vi "Turn Smother.vi"(2 "Ignore Deceleration":bool, 3 "Ignore Acceleration":bool, 4 "input cluster":T5={"Trajectory Data"=[], "Updated Waypoints"=[], {"Sample Period (s)"=0.0, "Limits"={"Velocity (fps)"=6.0, "Accel (fps^2)"=15.0, "Jerk (fps^3)"=150.0, "StoopidFast (fps)"=6.0}, "Conditions"={"vInitial (fps)"=0.0, "vFinal (fps)"=0.0}, "Angular Accelerations"={"Angular \nAccelerations"=[], "Override Limits?"=[]}}, "Array"=[]} {"?"."Limits"."StoopidFast (fps)" min=0.0; "?"."Limits"."Jerk (fps^3)" min=0.0 step=1.0; "?"."Limits"."Accel (fps^2)" min=0.0; "?"."Limits"."Velocity (fps)" min=0.0}) -> (0 "Velocities":dbl[](array[numeric]), 1 "Angular Accelerations":T1)   [LabVIEW 2019]
uses:
  Limits.ctl
  Command Stuff/Single Cmd Info.ctl
  <vilib>/picture/picture.llb/imagedata.ctl
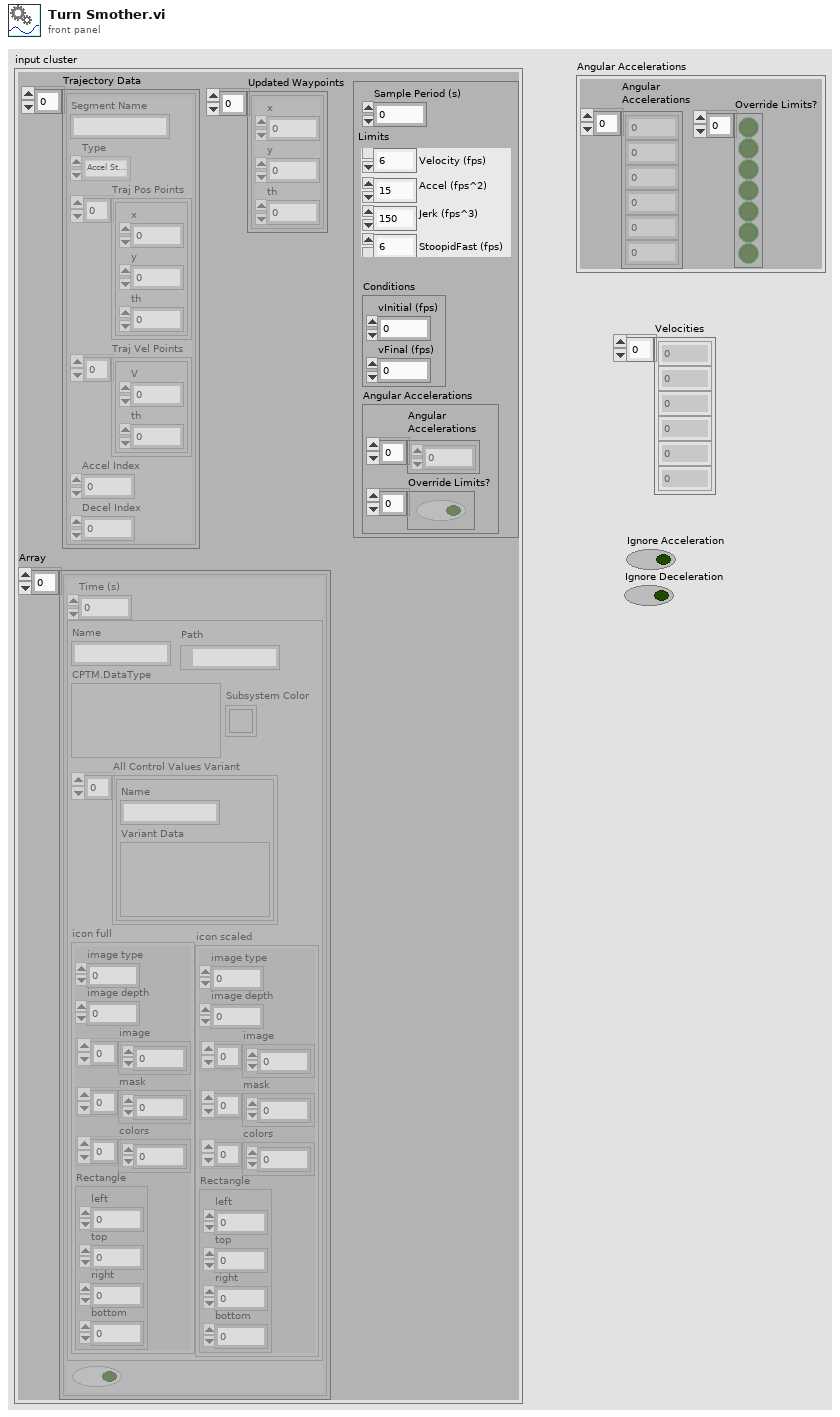
[diagram p1: front panel]
types:
  T1 = cluster{"Angular \nAccelerations":dbl[], "Override Limits?":bool[]}
  T2 = typedef "Limits.ctl" = cluster{"Velocity (fps)":dbl, "Accel (fps^2)":dbl, "Jerk (fps^3)":dbl, "StoopidFast (fps)":dbl}
  T3 = typedef "Single Cmd Info.ctl" = cluster{"Name":string, "CPTM.DataType":variant, "All Control Values Variant":cluster{"Name":string, "Variant Data":variant}[], "icon full":T4, "icon scaled":T4, "Path":path, "Subsystem Color":u32}
  T4 = typedef "imagedata.ctl" = cluster{"image type":i32, "image depth":i32, "image":u8[], "mask":u8[], "colors":u32[], "Rectangle":cluster{"left":i16, "top":i16, "right":i16, "bottom":i16}}
  T5 = cluster{"Trajectory Data":cluster{"Segment Name":string, "Type":enum16{"Accel Straight", "Const Straight", "Blend", "Circle"}, "Traj Pos Points":cluster{"x":dbl, "y":dbl, "th":dbl}[], "Traj Vel Points":cluster{"V":dbl, "th":dbl}[], "Accel Index":i32, "Decel Index":i32}[], "Updated Waypoints":cluster{"x":dbl, "y":dbl, "th":dbl}[], cluster{"Sample Period (s)":dbl, "Limits":T2, "Conditions":cluster{"vInitial (fps)":dbl, "vFinal (fps)":dbl}, "Angular Accelerations":cluster{"Angular \nAccelerations":dbl[], "Override Limits?":bool[]}}, "Array":cluster{"Time (s)":dbl, T3, bool}[]}
  T6 = cluster{"Segment Name":string, "Type":enum16{"Accel Straight", "Const Straight", "Blend", "Circle"}, "Traj Pos Points":cluster{"x":dbl, "y":dbl, "th":dbl}[], "Traj Vel Points":cluster{"V":dbl, "th":dbl}[], "Accel Index":i32, "Decel Index":i32}[]
  T7 = cluster{"Sample Period (s)":dbl, "Limits":T2, "Conditions":cluster{"vInitial (fps)":dbl, "vFinal (fps)":dbl}, "Angular Accelerations":cluster{"Angular \nAccelerations":dbl[], "Override Limits?":bool[]}}
  T8 = cluster{"vInitial (fps)":dbl, "vFinal (fps)":dbl}
  T9 = cluster{"Segment Name":string, "Type":enum16{"Accel Straight", "Const Straight", "Blend", "Circle"}, "Traj Pos Points":cluster{"x":dbl, "y":dbl, "th":dbl}[], "Traj Vel Points":cluster{"V":dbl, "th":dbl}[], "Accel Index":i32, "Decel Index":i32}
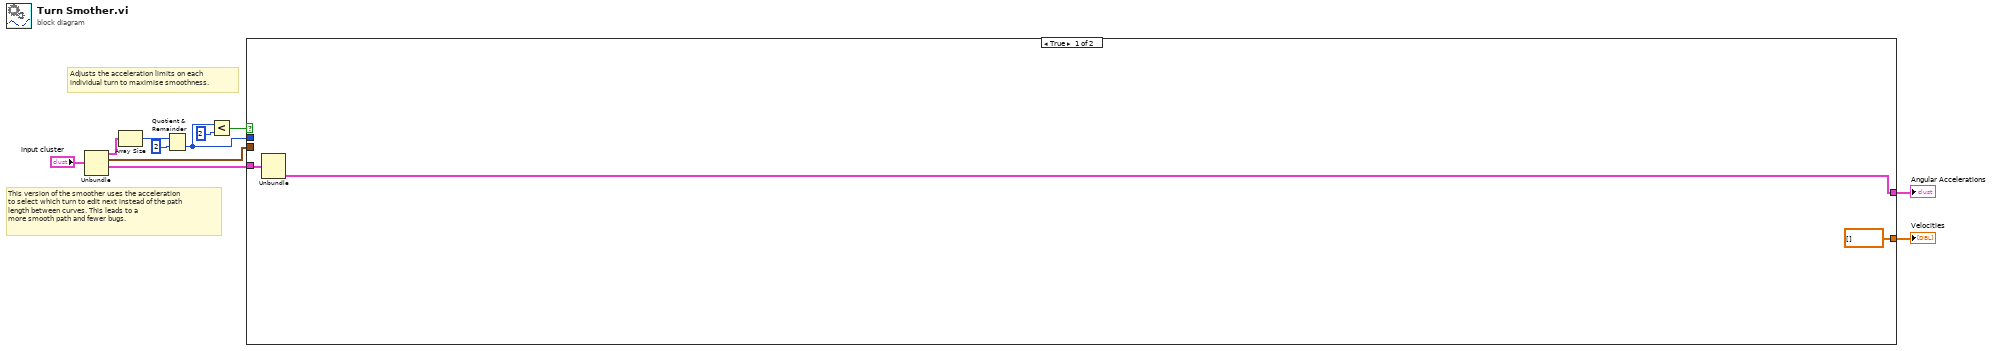
[diagram p0: block diagram]
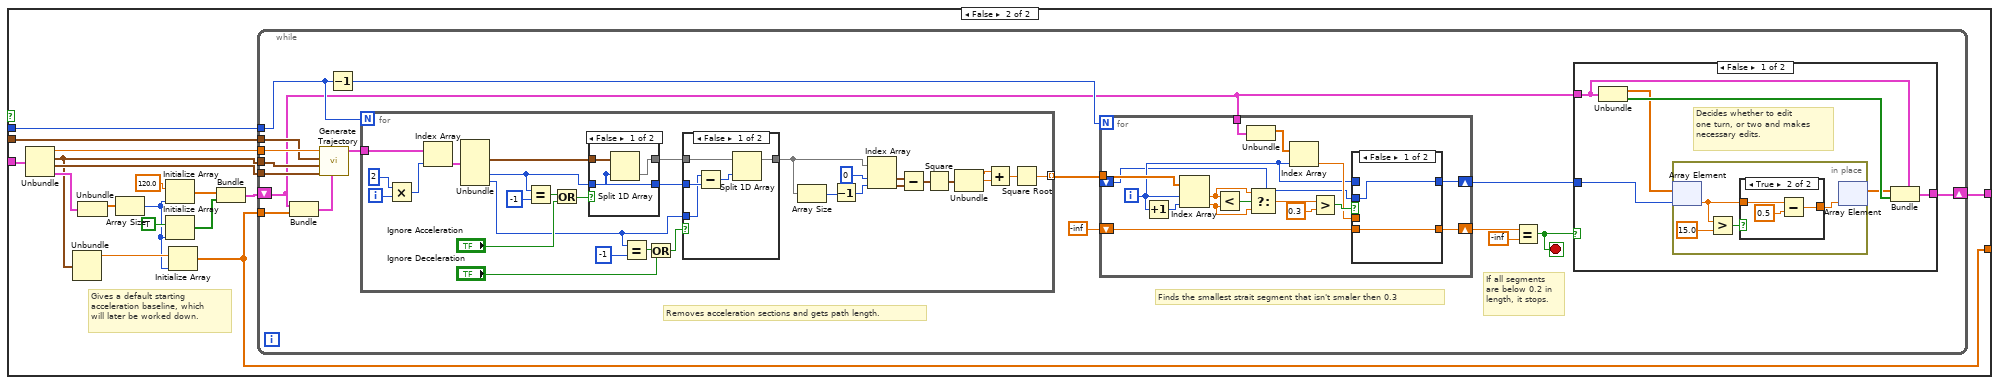
[diagram p2: hidden frame]
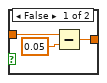
[diagram p3: hidden frame]
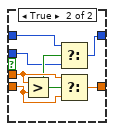
[diagram p7: hidden frame]
diagram:
  # "This version of the smoother uses the acceleration\nto select which turn to edit next instead of the path \nlength between curves. This leads to a \nmore smooth path and fewer bugs."
  # "Adjusts the acceleration limits on each \nindividual turn to maximise smoothness."
  n1 = Unbundle("input cluster") -> ("Trajectory Data"=w4:T6, "Updated Waypoints"=w3:cluster{"x":dbl, "y":dbl, "th":dbl}[], w5:T7)  [unwired: 1 out]
  n2 = Array Size(array=w4) -> (size(s)=w11:i32)
  n3 = Quotient & Remainder(x=w11, y=2) -> (floor(x/y)=w7:i32)  [unwired: 1 out]
  n4 = Less?(x=w7, y=2) -> (x < y?=w6:bool)
  n5 = case shown="True" w6 {
    tunnel: w7 -> [_ w29]
    tunnel: [w14 w28] -> w2
    tunnel: w5 -> [w13 w27]
    tunnel: w3 -> [_ w25]
    tunnel: [dbl[] [] w15] -> w1
    frame True {
      n6 = Unbundle(w13) -> ("Angular Accelerations"=w14:T1)  [unwired: 3 out]
    }
    frame False {
      # "Gives a default starting \nacceleration baseline, which\nwill later be worked down."
      n7 = Unbundle(w27) -> ("Sample Period (s)"=w26:dbl, "Limits"=w22:T2, "Conditions"=w24:T8, "Angular Accelerations"=w31:T1)
      n8 = Unbundle(w22) -> ("Velocity (fps)"=w23:dbl)  [unwired: 3 out]
      n9 = Unbundle(w31) -> ("Angular \nAccelerations"=w16:dbl[])  [unwired: 1 out]
      n10 = Array Size(array=w16) -> (size(s)=w18:i32)
      n11 = Initialize Array(120.0, w18) -> (w17:dbl[])
      n12 = Initialize Array(TRUE, w18) -> (w20:bool[])
      n13 = Initialize Array(w23, w18) -> (w15:dbl[])
      n14 = Bundle(w17, w20) -> (w30:cluster{dbl[], bool[]})  [unwired: 1 in]
      n15 = while {
        shift-right: [w46] -> w28
        shift-left: w30 -> [w34]
        tunnel: w29 -> [w43]
        tunnel: w26 -> [w41]
        tunnel: w25 -> [w40]
        tunnel: w22 -> [w39]
        tunnel: w24 -> [w38]
        tunnel: w15 -> [w33]
        stop <- w48 stop-if-true
        # "If all segments\nare below 0.2 in\nlength, it stops."
        # "Removes acceleration sections and gets path length."
        # "Finds the smallest strait segment that isn't smaler then 0.3"
        n16 = Bundle(w34, w33) -> (w32:cluster{cluster{dbl[], bool[]}, dbl[]})  [unwired: 1 in]
        n17 = call "Generate Trajectory.vi"("Overrides"=w32, "Conditions"=w38, "Limits"=w39, "WayPoints"=w40, "Sample Period (s)"=w41) -> ("Trajectory Data"=w42:T6)  [unwired: 2 in, 4 out]
        n18 = Decrement(x=w43) -> (x-1=w44:i32)
        n19 = for {
          N: w43 -> [_]
          tunnel: w42 -> [w93]
          tunnel: [w83] -> w45 mode=indexing
          i -> [w95]
          n20 = Multiply(x=2, y=w95) -> (x*y=w92:i32)
          n21 = Index Array(array=w93, index=w92) -> (element=w91:T9)
          n22 = Unbundle(w91) -> ("Traj Pos Points"=w84:cluster{"x":dbl, "y":dbl, "th":dbl}[], "Accel Index"=w80:i32, "Decel Index"=w73:i32)  [unwired: 3 out]
          n23 = Equal?(x=w80, y=-1) -> (x = y?=w81:bool)
          n24 = Or(x=w81, y="Ignore Acceleration") -> (x .or. y?=w79:bool)
          n25 = case shown="False" w79 {
            tunnel: w84 -> [w104 w105]
            tunnel: [w103 w105] -> w90
            tunnel: [w102 _] -> w89
            tunnel: w80 -> [w102 _]
            frame False {
              n26 = Split 1D Array(array=w104, index=w102) -> (second subarray=w103:cluster{"x":dbl, "y":dbl, "th":dbl}[])  [unwired: 1 out]
            }
            frame True {
            }
          }
          n27 = Equal?(x=w73, y=-1) -> (x = y?=w76:bool)
          n28 = Or(x=w76, y="Ignore Deceleration") -> (x .or. y?=w74:bool)
          n29 = case shown="False" w74 {
            tunnel: w90 -> [w100 w101]
            tunnel: [w99 w101] -> w87
            tunnel: w89 -> [w98 _]
            tunnel: w73 -> [w96 _]
            frame False {
              n30 = Subtract(x=w96, y=w98) -> (x-y=w97:i32)
              n31 = Split 1D Array(array=w100, index=w97) -> (first subarray=w99:cluster{"x":dbl, "y":dbl, "th":dbl}[])  [unwired: 1 out]
            }
            frame True {
            }
          }
          n32 = Array Size(array=w87) -> (size(s)=w86:i32)
          n33 = Decrement(x=w86) -> (x-1=w85:i32)
          n34 = Index Array(array=w87, index #1=0 ("index"), index #2=w85) -> (element #1=w72:cluster{"x":dbl, "y":dbl, "th":dbl}, element #2=w71:cluster{"x":dbl, "y":dbl, "th":dbl})
          n35 = Subtract(x=w72, y=w71) -> (x-y=w70:cluster{"x":dbl, "y":dbl, "th":dbl})
          n36 = Square(x=w70) -> (x^2=w69:cluster{"x":dbl, "y":dbl, "th":dbl})
          n37 = Unbundle(w69) -> ("x"=w67:dbl, "y"=w68:dbl)  [unwired: 1 out]
          n38 = Add(x=w67, y=w68) -> (x+y=w66:dbl)
          n39 = Square Root(x=w66) -> (sqrt(x)=w83:dbl)
        }
        n40 = for {
          N: w44 -> [_]
          tunnel: w45 -> [w121]
          shift-right: [w116] -> w47
          shift-left: -inf -> [w115]
          tunnel: w34 -> [w111]
          shift-right: [w107] -> w35
          shift-left: _ -> [w106]
          i -> [w108]
          n41 = Increment(x=w108) -> (x+1=w120:i32)
          n42 = Index Array(array=w121, index #1=w108, index #2=w120) -> (element #1=w117:dbl, element #2=w118:dbl)
          n43 = Less?(x=w117, y=w118) -> (x < y?=w119:bool)
          n44 = Unbundle(w111) -> (w110:dbl[])  [unwired: 1 out]
          n45 = Select(t=w117, s=w119, f=w118) -> (s? t:f=w113:dbl)
          n46 = Index Array(array=w110, index=w108) -> (element=w109:dbl)
          n47 = Greater?(x=w113, y=0.3) -> (0:w114:bool)
          n48 = case shown="False" w114 {
            tunnel: [w123 w130] -> w116
            tunnel: w115 -> [w123 w129]
            tunnel: w109 -> [_ w128]
            tunnel: w108 -> [_ w126]
            tunnel: [w122 w124] -> w107
            tunnel: w106 -> [w122 w125]
            frame False {
            }
            frame True {
              n49 = Greater?(x=w128, y=w129) -> (0:w127:bool)
              n50 = Select(t=w126, s=w127, f=w125) -> (s? t:f=w124:i32)
              n51 = Select(t=w128, s=w127, f=w129) -> (s? t:f=w130:dbl)
            }
          }
        }
        n52 = Equal?(x=w47, y=-inf) -> (x = y?=w48:bool)
        n53 = case shown="False" w48 {
          tunnel: w34 -> [w53 w65]
          tunnel: [w52 w65] -> w46
          tunnel: w35 -> [w49 _]
          frame False {
            # "Decides whether to edit\none turn, or two and makes\nnecessary edits."
            n54 = Unbundle(w53) -> (w51:dbl[], w54:bool[])
            n55 = in-place {
              n56 = in-place-array #1(w51, w49) -> (w55:dbl)
              n57 = Greater?(x=w55, y=15.0) -> (0:w56:bool)
              n58 = case shown="True" w56 {
                tunnel: [w60 w63] -> w58
                tunnel: w55 -> [w61 w62]
                frame False {
                  n59 = Subtract(x=w61, y=0.05) -> (x-y=w60:dbl)
                }
                frame True {
                  n60 = Subtract(x=w62, y=0.5) -> (x-y=w63:dbl)
                }
              }
              n61 = in-place-array #1(w58) -> (w50:dbl[])  [unwired: 1 out]
            }
            n62 = Bundle(cluster=w53, w50, w54) -> (w52:cluster{dbl[], bool[]})
          }
          frame True {
          }
        }
      }
    }
  }
  "Angular Accelerations" <- w2
  "Velocities" <- w1
